vi "Construct Sequence Variable Igor String.vi"(10 "Current index":i32, 11 "VariableManagerRef":refnum<vi>) -> (3 "Igor Instruction String":string[](array[string]))   [LabVIEW 2013]
uses:
  VariableManagerCodes/VariableManager/VariableManager.lvclass
  VariableManagerCodes/Variable/Variable.lvclass
  VariableManagerCodes/VariableValue/VariableValue.lvclass
  VariableManagerCodes/API/VariableManagerAPI.lvlib
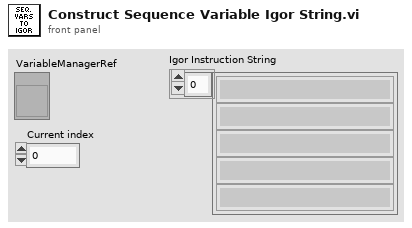
[diagram p1: front panel]
types:
  T1 = enum16{"Floating point", "Scientific SI", "Automatic SI", "SI notation"}
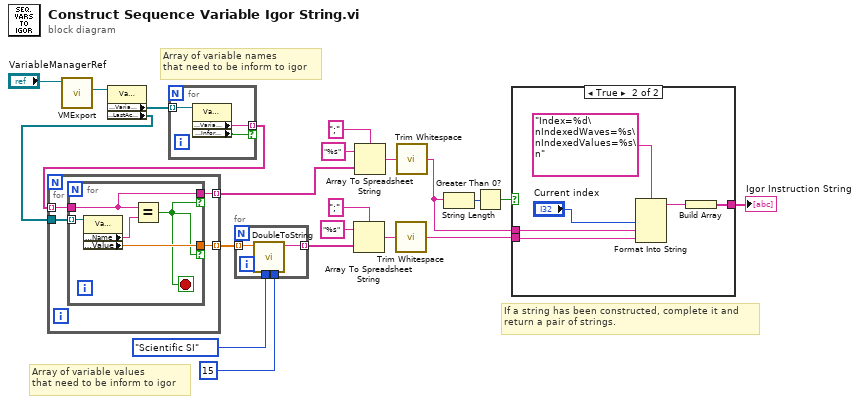
[diagram p0: block diagram]
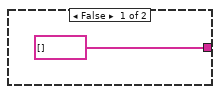
[diagram p2: hidden frame]
diagram:
  # "Array of variable values\nthat need to be inform to igor"
  # "Array of variable names\nthat need to be inform to igor"
  # "If a string has been constructed, complete it and\nreturn a pair of strings."
  n1 = call "VMExport.vi"("VariableManagerRef in"="VariableManagerRef") -> ("VariableManagerExportCopy"=w17:refnum<class "VariableManager.lvclass">)  [unwired: 8 in, 2 out]
  n2 = property class="VariableManager.lvclass"(reference=w17) -> ("Accessors:Variables"=w16:refnum<class "Variable.lvclass">[], "Accessors:LastAcquireValues"=w15:refnum<class "VariableValue.lvclass">[])  [unwired: 1 in, 2 out]
  n3 = for {
    tunnel: w16 -> [w24] mode=indexing
    tunnel: [w22] -> w14 mode=indexing if=w23
    n4 = property class="Variable.lvclass"(reference=w24) -> ("Accessors:VariableName"=w22:string, "Accessors:InformIgor"=w23:bool)  [unwired: 1 in, 2 out]
  }
  n5 = for {
    tunnel: w14 -> [w27] mode=indexing
    tunnel: w15 -> [w28]
    tunnel: [w26] -> w11 mode=indexing
    tunnel: [w25] -> w1 mode=indexing
    n6 = for {
      tunnel: w28 -> [w33] mode=indexing
      tunnel: w27 -> [w30]
      tunnel: [w31] -> w26 if=w29
      tunnel: [w30] -> w25 if=w29
      stop <- w29 stop-if-true
      n7 = property class="VariableValue.lvclass"(reference=w33) -> ("Accessors:Name"=w32:string, "Accessors:Value"=w31:dbl)  [unwired: 1 in, 2 out]
      n8 = Equal?(x=w30, y=w32) -> (x = y?=w29:bool)
    }
  }
  n9 = for {
    tunnel: w11 -> [w37] mode=indexing
    tunnel: T1."Scientific SI" ("Format (SI notation)") -> [w36]
    tunnel: u32 15 ("SignificantDigits (8)") -> [w35]
    tunnel: [w34] -> w6 mode=indexing
    n10 = call "DoubleToString.vi"("SignificantDigits (8)"=w35, "Format (SI notation)"=w36, "Double"=w37) -> ("String"=w34:string)  [unwired: 8 in]
  }
  n11 = Array To Spreadsheet String(delimiter (Tab)=";", array=w6, 3:"%s" ("format string")) -> (spreadsheet string=w3:string)
  n12 = Array To Spreadsheet String(delimiter (Tab)=";", array=w1, 3:"%s" ("format string")) -> (spreadsheet string=w5:string)
  n13 = call <vilib>:"Trim Whitespace.vi"("string"=w3) -> ("trimmed string"=w2:string)  [unwired: 1 in]
  n14 = call <vilib>:"Trim Whitespace.vi"("string"=w5) -> ("trimmed string"=w4:string)  [unwired: 1 in]
  n15 = String Length(string=w4) -> (length=w20:i32)
  n16 = Greater Than 0?(x=w20) -> (x > 0?=w19:bool)
  n17 = case shown="True" w19 {
    tunnel: w4 -> [_ w43]
    tunnel: w2 -> [_ w42]
    tunnel: [string[] [] w39] -> w21
    frame False {
    }
    frame True {
      n18 = Format Into String(format string="Index=%d\nIndexedWaves=%s\nIndexedValues=%s\n", "Current index", w43, w42) -> (resulting string=w40:string)  [unwired: 2 in, 1 out]
      n19 = Build Array(w40) -> (w39:string[])
    }
  }
  "Igor Instruction String" <- w21
